vi "Utility - Determine dx-dy from distance and slope.vi"(10 "Slope (dy/dx)":dbl, 11 "Distance= r":dbl) -> (2 "dy":dbl, 3 "dx":dbl)   [LabVIEW 2012]
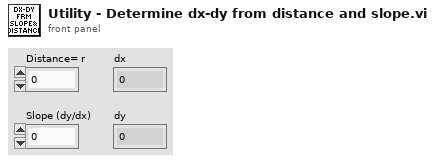
[diagram p1: front panel]
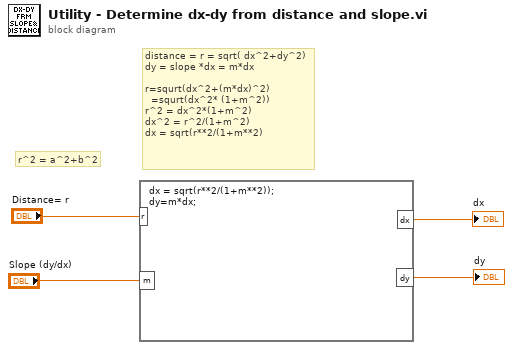
[diagram p0: block diagram]
diagram:
  # "r^2 = a^2+b^2"
  # "distance = r = sqrt( dx^2+dy^2)\ndy = slope *dx = m*dx\n\nr=squrt(dx^2+(m*dx)^2) \n  =squrt(dx^2* (1+m^2))\nr^2 = dx^2*(1+m^2)\ndx^2 = r^2/(1+m^2)\ndx = sqrt(r**2/(1+m**2)"
  n1 = formula code="dx = sqrt(r**2/(1+m**2));\ndy=m*dx;"("r"="Distance= r", "m"="Slope (dy/dx)") -> ("dx"=→"dx":dbl, "dy"=→"dy":dbl)
